vi "Even Bit Extractor.vi"() -> ()   [LabVIEW 2026]
panel:
  out "Even Bits":i8
  in  "loop Index":i8
  in  "Input PN sequence":i8[](array[numeric])
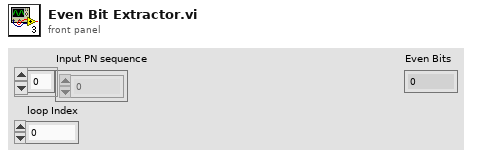
[diagram p1: front panel]
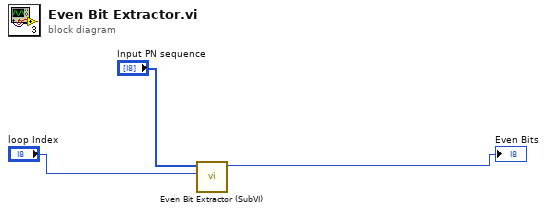
[diagram p0: block diagram]
diagram:
  n1 = call "Even Bit Extractor (SubVI).vi"("loop Index"="loop Index", "Input PN sequence"="Input PN sequence") -> ("Even Bits"=→"Even Bits":i8)  [unwired: 9 in]
